vi "Stop Core.vi"(10 "final error code":i32, 11 "MediatorBusMonitor in":refnum<class "MediatorBusMonitor.lvclass">) -> (3 "MediatorBusMonitor out":refnum<class "MediatorBusMonitor.lvclass">)   [LabVIEW 2017, in "Mediator.lvlib" / "MediatorBusMonitor.lvclass"]
doc: "(<B>Filename</B>: Actor Framework.lvlib:Actor.lvclass:Stop Core.vi)\n\nDefines what the actor does before it stops. Use the <B>final error code</B> input to determine whether the actor shut down in response to an error.\n\nBy default, this method does nothing. A descendant class may override it to define behavior, such as shutting down any processes the actor initiated in its override of the Actor Core method.\n\n<License>\nCopyright © 2017 Composed Systems, LLC | All rights reserved\nwww.composed.io\n\nAuthor: Ethan Stern <ethan.stern@composed.io>\n\nThis software is provided \"AS IS\" WITHOUT WARRANTIES, either express or implied, AND IS FOR EDUCATIONAL PURPOSES ONLY.\n</License>"
uses:
  MediatorBusMonitor.lvclass
  MediatorBusMonitor.lvclass/MediatorBusMonitor.ctl
  IMediator/IMediatorBusMonitor/MediatorBusMonitor/IMediatorBusMonitor.lvclass
  gpm_packages/@cs/lookup-table/Source/LookupTable/LookupTable.lvclass
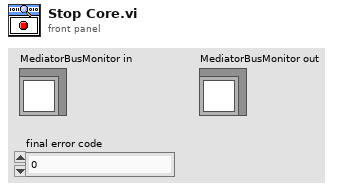
[diagram p1: front panel]
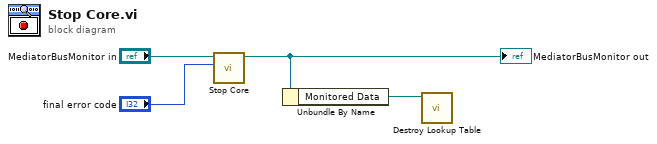
[diagram p0: block diagram]
diagram:
  n1 = call-parent "Stop Core.vi"("final error code"="final error code", "IViewable in"="MediatorBusMonitor in") -> ("IViewable out"=w2:refnum<class "MediatorBusMonitor.lvclass">)  [unwired: 9 in]
  "MediatorBusMonitor out" <- w2
  n2 = Unbundle By Name(w2) -> ("Monitored Data"=w1:refnum<data-value>)
  n3 = call "Destroy Lookup Table.vi"("LookupTable Reference"=w1) -> ()  [unwired: 10 in, 1 out]
